vi "Channel Interface.vi"(8 "error in (no error)":errorcluster, 11 "Node Ptr":T1 format="%.0x") -> (0 "error out":errorcluster)   [LabVIEW 2017, in "ALMA_10201-10401_O2SensorSim System Explorer.lvlib"]
uses:
  ALMA_10201-10401_O2SensorSim System Explorer.lvlib
  <vilib>/NI Veristand/Custom Device API/Custom Device Item Ref.ctl
  <vilib>/NI Veristand/Custom Device API/Custom Device Channel Type.ctl
  Shared/Constants.vi
  <vilib>/NI Veristand/Custom Device API/Get Item Property (String).vi
  <vilib>/NI Veristand/Custom Device Tools/Custom Device Utility Library/NI VeriStand - Search for Item by Name.vi
  <vilib>/NI Veristand/Custom Device API/Custom Device API.lvlib
  <vilib>/NI Veristand/Custom Device Tools/Custom Device Utility Library/Custom Device Utility Library.lvlib
  Shared/ALMA_10201-10401_O2SensorSim Shared.lvlib
panel:
  out "Documentation":string
  in  "Default Value":dbl
  out "Access":i32(ring) items=["None", "Read Only", "Write Only", "Read/Write"]
  out "SLSC Information":string
  in  "Header":cluster{"Section Name":string}={"Section Name"="Custom Device Item Settings"}
  out "Description":string
  out "Name":string
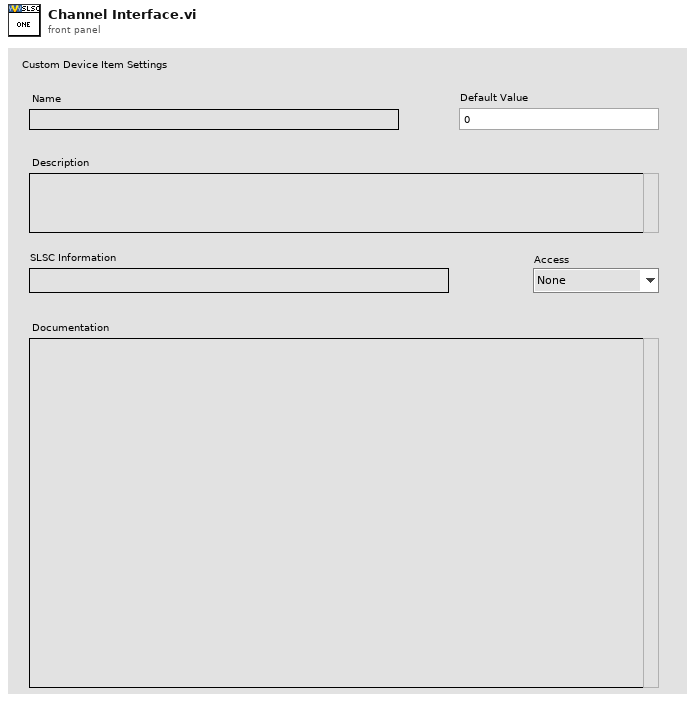
[diagram p1: front panel]
types:
  T1 = typedef "Custom Device API.lvlib/Custom Device Item Ref.ctl" = u64
  T2 = typedef "Custom Device API.lvlib/Custom Device Channel Type.ctl" = enum16{"Input", "Output"}
  T3 = enum8{"Enabled", "Disabled", "Disabled and Grayed Out"}
  T4 = typedef "Custom Device API.lvlib/Custom Device Item Info.ctl" = cluster{"Name":string, "Is Channel":bool, "GUID":string, "Is Waveform":bool}
  T5 = typedef "Custom Device API.lvlib/Custom Device Channel.ctl" = cluster{"Type":T2, "Units":string, "Default Value":dbl, "Faultable":bool, "Scalable":bool}
  T6 = typedef "Custom Device API.lvlib/Custom Device Commands.ctl" = enum16{"Default", "Item renamed", "Shutdown", "Dynamic button pressed"}
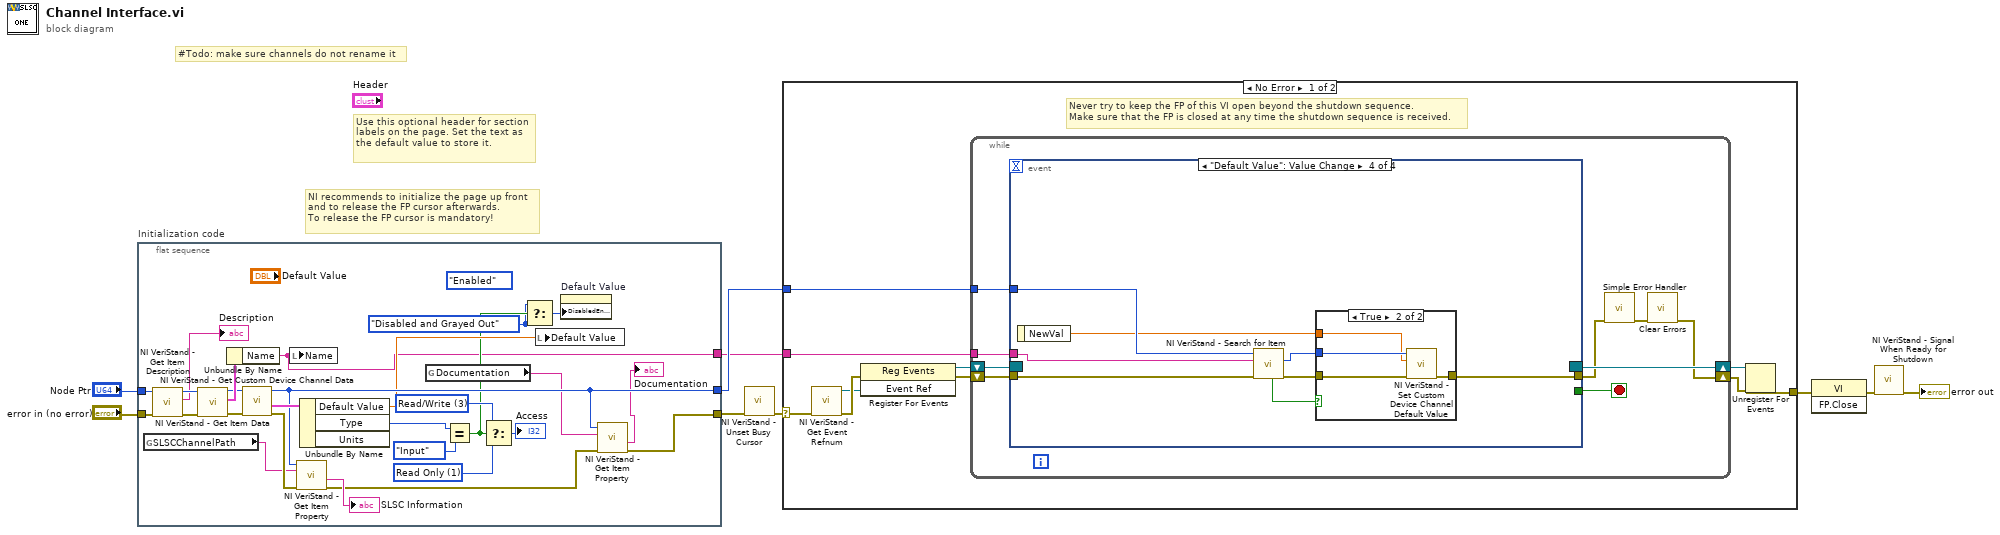
[diagram p0: block diagram]
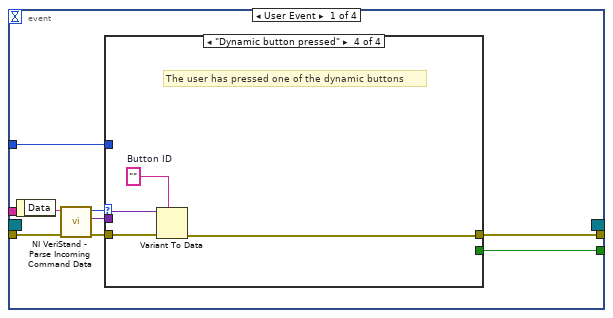
[diagram p2: hidden frame]
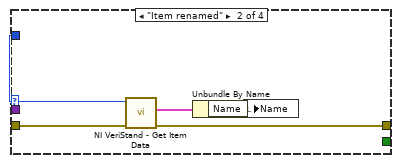
[diagram p4: hidden frame]
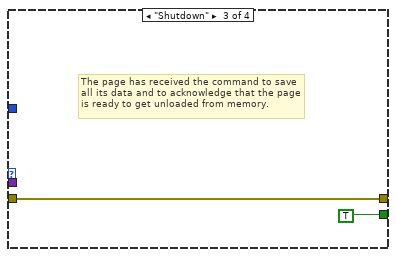
[diagram p5: hidden frame]
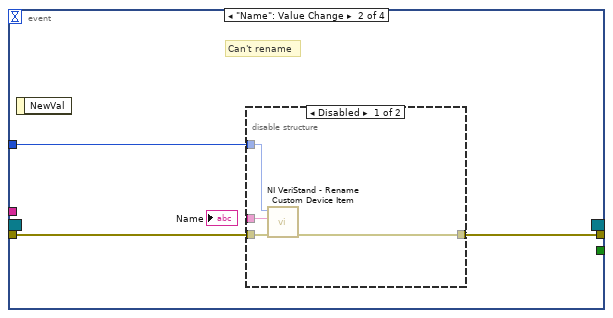
[diagram p6: hidden frame]
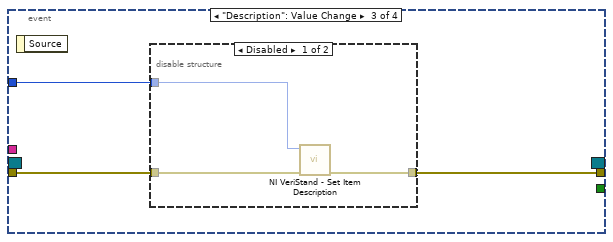
[diagram p8: hidden frame]
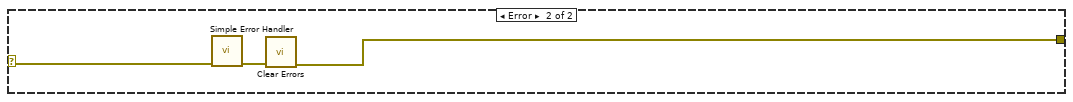
[diagram p11: hidden frame]
diagram:
  # "#Todo: make sure channels do not rename it"
  # "Use this optional header for section labels on the page. Set the text as the default value to store it."
  # "NI recommends to initialize the page up front\nand to release the FP cursor afterwards.\nTo release the FP cursor is mandatory!"
  n1 = flat-sequence "Initialization code" {
    tunnel: "error in (no error)" -> [w35]
    tunnel: "Node Ptr" -> [w34]
    tunnel: [w18] -> w5
    tunnel: [w21] -> w2
    tunnel: [w14] -> w1
    frame #0 {
      w12 = T3."Disabled and Grayed Out" ("Disabled")
      (unwired) T3."Enabled" ("Disabled")
      w31 = 1 items=["None", "Read Only", "Write Only", "Read/Write"] ("Access")
      w30 = 3 items=["None", "Read Only", "Write Only", "Read/Write"] ("Access")
      n2 = global read "Constants.vi" "SLSCChannelPath"() -> (w10:string)
      n3 = call <vilib>:"NI VeriStand - Get Item Description.vi"("error in (no error)"=w35, "Item Ref in"=w34) -> ("error out"=w33:errorcluster, "Description"=→"Description":string, "Item Ref out"=w36:T1)  [unwired: 7 out]
      n4 = call <vilib>:"NI VeriStand - Get Item Data.vi"("error in (no error)"=w33, "Item Ref in"=w36) -> ("error out"=w22:errorcluster, "Item Info"=w32:T4, "Item Ref out"=w23:T1)  [unwired: 7 out]
      n5 = Unbundle By Name(w32) -> ("Name"=w14:string)
      n6 = call <vilib>:"NI VeriStand - Get Custom Device Channel Data.vi"("error in (no error)"=w22, "Channel Ref in"=w23) -> ("error out"=w26:errorcluster, "Channel"=w24:T5, "Channel Ref out"=w21:T1)  [unwired: 4 in, 3 out]
      n7 = local write "Name"(w14) -> ()
      n8 = call-poly <vilib>:"NI VeriStand - Get Item Property.vi"("error in (no error)"=w26, "Property Name"=w10, "Item Ref in"=w21) -> ("error out"=w20:errorcluster, "Value"=→"SLSC Information":string)  [unwired: 5 in, 2 out]
      n9 = Unbundle By Name(w24) -> ("Default Value"=w16:dbl, "Type"=w27:T2)  [unwired: 1 out]
      n10 = global read "Constants.vi" "Documentation"() -> (w11:string)
      n11 = Equal?(x=w27, y=Custom_Device_Channel_Type."Input") -> (x = y?=w15:bool)
      n12 = Select(t=w30, s=w15, f=w31) -> (s? t:f=→"Access":i32)
      n13 = Select(t=w12, s=w15, f=w12) -> (s? t:f=w13:T3)
      n14 = local write "Default Value"(w16) -> ()
      n15 = property on="Default Value" class="DigNum (strict)"("DisabledEnum"=w13) -> ()  [unwired: 2 in, 2 out]
      n16 = call-poly <vilib>:"NI VeriStand - Get Item Property.vi"("error in (no error)"=w20, "Property Name"=w11, "Item Ref in"=w21) -> ("error out"=w18:errorcluster, "Value"=→"Documentation":string)  [unwired: 5 in, 2 out]
    }
  }
  n17 = call <vilib>:"NI VeriStand - Unset Busy Cursor.vi"("error in (no error)"=w5) -> ("error out"=w4:errorcluster)  [unwired: 10 out]
  n18 = case shown="No Error" w4 {
    selector: w4 -> [w38 w104]
    tunnel: [w43 w102] -> w9
    tunnel: w2 -> [w39 _]
    tunnel: w1 -> [w37 _]
    frame No Error {
      # "Never try to keep the FP of this VI open beyond the shutdown sequence.\nMake sure that the FP is closed at any time the shutdown sequence is received."
      n19 = call <vilib>:"NI VeriStand - Get Event Refnum.vi"("error in (no error)"=w38) -> ("error out"=w46:errorcluster, "Event Ref"=w42:refnum<user-event>)  [unwired: 9 out]
      n20 = register-events(error in=w46, w42) -> (reference out=w40:refnum<event-registration>, error out=w41:errorcluster)  [unwired: 1 in]
      n21 = while {
        tunnel: w39 -> [w51]
        shift-right: [w48] -> w44
        shift-left: w41 -> [w54]
        shift-right: [w55] -> w45
        shift-left: w40 -> [w53]
        tunnel: w37 -> [w47]
        stop <- w52 stop-if-true
        n22 = event shown="[3] \"Default Value\": Value Change" {
          selector: w53 -> [_ _ _ _]
          dyn-events: [_ _ _ _] -> w55
          timeout: _ -> [_ _ _ _]
          tunnel: w54 -> [w63 w78 w84 w93]
          tunnel: [w59 _ _ _] -> w52
          tunnel: [w58 w77 w83 w91] -> w50
          tunnel: w51 -> [w57 w76 w85 w96]
          tunnel: w47 -> [_ _ _ w90]
          event User Event {
            n23 = event-data() -> ("Data"=w62:string)  [unwired: 1 out]
            n24 = call <vilib>:"NI VeriStand - Parse Incoming Command Data.vi"("error in (no error)"=w63, "Incoming data"=w62) -> ("error out"=w61:errorcluster, "Outgoing data"=w56:variant, "Action"=w60:T6)  [unwired: 7 out]
            n25 = case shown="\"Dynamic button pressed\"" w60 {
              tunnel: w61 -> [w64 w69 w70 w75]
              tunnel: [_ _ TRUE _] -> w59
              tunnel: [w64 w66 w70 w72] -> w58
              tunnel: w57 -> [_ w68 _ _]
              tunnel: w56 -> [_ _ _ w74]
              frame "Default", Default {
              }
              frame "Item renamed" {
                n26 = call <vilib>:"NI VeriStand - Get Item Data.vi"("error in (no error)"=w69, "Item Ref in"=w68) -> ("error out"=w66:errorcluster, "Item Info"=w67:T4)  [unwired: 8 out]
                n27 = Unbundle By Name(w67) -> ("Name"=w65:string)
                n28 = local write "Name"(w65) -> ()
              }
              frame "Shutdown" {
                # "The page has received the command to save all its data and to acknowledge that the page is ready to get unloaded from memory."
              }
              frame "Dynamic button pressed" {
                w73 = ""  # Button ID
                # "The user has pressed one of the dynamic buttons"
                n29 = Variant To Data(error in=w75, type=w73, Variant=w74) -> (error out=w72:errorcluster)  [unwired: 1 out]
              }
            }
          }
          event "Name": Value Change {
            # "Can't rename"
            n30 = event-data() -> ()  [unwired: 2 out]
            n31 = disable-structure shown="Disabled" {
              disable-tunnel: w78 -> [w82 _]
              disable-tunnel: [w81 _] -> w77
              disable-tunnel: w76 -> [w80 _]
              disable-tunnel: _ -> [w79 _]
              frame Disabled {
                n32 = call <vilib>:"NI VeriStand - Rename Custom Device Item.vi"("error in (no error)"=w82, "New Name"=w79, "Item Ref in"=w80) -> ("error out"=w81:errorcluster)  [unwired: 1 in, 7 out]
              }
              frame Enabled {
              }
            }
          }
          event "Description": Value Change {
            n33 = event-data() -> ()  [unwired: 2 out]
            n34 = disable-structure shown="Disabled" {
              disable-tunnel: w85 -> [w88 _]
              disable-tunnel: w84 -> [w87 _]
              disable-tunnel: [w86 _] -> w83
              frame Disabled {
                n35 = call <vilib>:"NI VeriStand - Set Item Description.vi"("error in (no error)"=w87, "Item Ref in"=w88) -> ("error out"=w86:errorcluster)  [unwired: 1 in, 8 out]
              }
              frame Enabled {
              }
            }
          }
          event "Default Value": Value Change {
            n36 = event-data() -> ("NewVal"=w94:dbl)  [unwired: 1 out]
            n37 = call-poly <vilib>:"NI VeriStand - Search for Item.vi"("error in"=w93, "Item Name"=w90, "Section Ref in"=w96) -> ("error out"=w92:errorcluster, "Item Ref"=w95:T1, "Found"=w89:bool)  [unwired: 5 in, 1 out]
            n38 = case shown="True" w89 {
              tunnel: w95 -> [_ w101]
              tunnel: w94 -> [_ w100]
              tunnel: w92 -> [w97 w99]
              tunnel: [w97 w98] -> w91
              frame False {
              }
              frame True {
                n39 = call <vilib>:"NI VeriStand - Set Custom Device Channel Default Value.vi"("error in (no error)"=w99, "Default Value"=w100, "Channel Ref in"=w101) -> ("error out"=w98:errorcluster)  [unwired: 7 in, 1 out]
              }
            }
          }
        }
        n40 = call <vilib>:"Simple Error Handler.vi"("error in (no error)"=w50) -> ("error out"=w49:errorcluster)  [unwired: 1 in, 7 out]
        n41 = call <vilib>:"Clear Errors.vi"("error in (no error)"=w49) -> ("error out"=w48:errorcluster)  [unwired: 1 in, 5 out]
      }
      n42 = Unregister For Events(event registration refnum=w45, error in=w44) -> (error out=w43:errorcluster)
    }
    frame Error {
      n43 = call <vilib>:"Simple Error Handler.vi"("error in (no error)"=w104) -> ("error out"=w103:errorcluster)  [unwired: 1 in, 7 out]
      n44 = call <vilib>:"Clear Errors.vi"("error in (no error)"=w103) -> ("error out"=w102:errorcluster)  [unwired: 1 in, 5 out]
    }
  }
  n45 = invoke class="VI" method="FP.Close"(error in=w9) -> (error out=w8:errorcluster)  [unwired: 2 in, 2 out]
  n46 = call <vilib>:"NI VeriStand - Signal When Ready for Shutdown.vi"("error in (no error)"=w8) -> ("error out"=→"error out":errorcluster)  [unwired: 10 out]
